vi "Is Point In Shape(1).vi"(8 "error in (no error)":errorcluster, 10 "Point":cluster{"Horizontal":i32, "Vertical":i32}, 11 "Rectangle in":refnum<class "Rectangle.lvclass">) -> (0 "error out":errorcluster, 2 "Point In Shape?":bool, 3 "Rectangle out":refnum<class "Rectangle.lvclass">)   [LabVIEW 2015, in "Rectangle.lvclass"]
uses:
  Rectangle.lvclass
  Interfaces/Shape/Shape.lvclass/Shape.ctl
  Interfaces/Shape/Shape.lvclass
panel:
  # "NOTICE -- YOU MUST LEAVE THIS NOTICE IN PLACE.\n\nCopyright (c) 2017, LIANG LIU Shawn.Liu.cn@gmail.com\nAll rights reserved.\n\nRedistribution and use in source and binary forms, with or without modification, are permitted provided that the following conditions are met:\n-Redistributions of source code must retain the above copyright notice, this list of conditions and the following disclaimer.\n-Redistributions in binary form must reproduce the above copyright notice, this list of conditions and the following disclaimer in the documentation and/or other materials provided with the distribution.\n-Neither the name of the eLp nor the names of its contributors may be used to endorse or promote products derived from this software without specific prior written permission.\n\nTHIS SOFTWARE IS PROVIDED BY THE COPYRIGHT HOLDERS AND CONTRIBUTORS \"AS IS\" AND ANY EXPRESS OR IMPLIED WARRANTIES, INCLUDING, BUT NOT LIMITED TO, THE IMPLIED WARRANTIES OF MERCHANTABILITY AND FITNESS FOR A PARTICULAR PURPOSE ARE DISCLAIMED. IN NO EVENT SHALL THE COPYRIGHT HOLDER OR CONTRIBUTORS BE LIABLE FOR ANY DIRECT, INDIRECT, INCIDENTAL, SPECIAL, EXEMPLARY, OR CONSEQUENTIAL DAMAGES (INCLUDING, BUT NOT LIMITED TO, PROCUREMENT OF SUBSTITUTE GOODS OR SERVICES; LOSS OF USE, DATA, OR PROFITS; OR BUSINESS INTERRUPTION) HOWEVER CAUSED AND ON ANY THEORY OF LIABILITY, WHETHER IN CONTRACT, STRICT LIABILITY, OR TORT (INCLUDING NEGLIGENCE OR OTHERWISE) ARISING IN ANY WAY OUT OF THE USE OF THIS SOFTWARE, EVEN IF ADVISED OF THE POSSIBILITY OF SUCH DAMAGE."
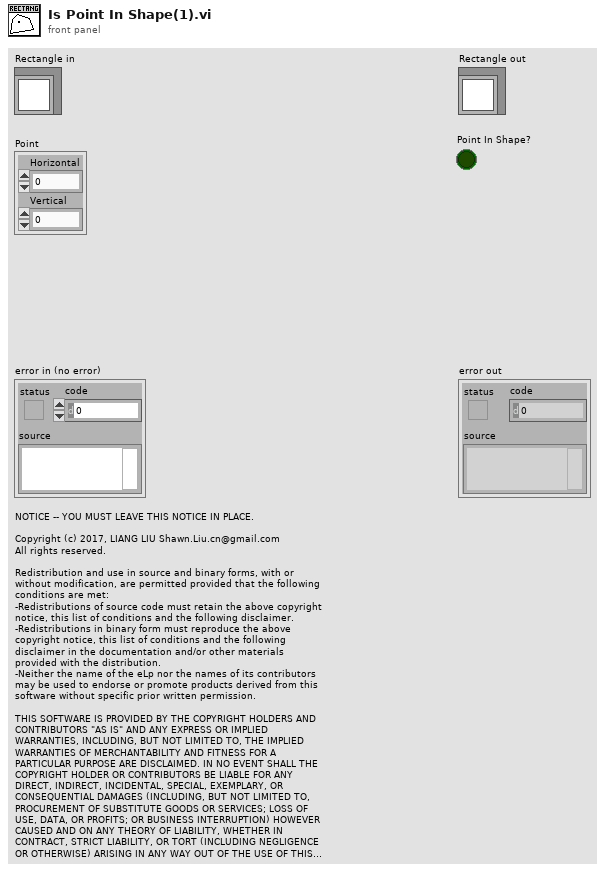
[diagram p1: front panel]
types:
  T1 = cluster{"left":i16, "top":i16, "right":i16, "bottom":i16}
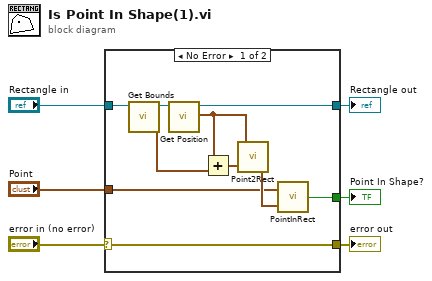
[diagram p0: block diagram]
diagram:
  n1 = case shown="No Error" "error in (no error)" {
    selector: "error in (no error)" -> [w16 w18]
    tunnel: "Rectangle in" -> [w15 w17]
    tunnel: [w13 w17] -> w4
    tunnel: "Point" -> [w8 _]
    tunnel: [w7 _] -> w2
    tunnel: [w16 w18] -> w1
    frame No Error {
      n2 = call "Get Bounds.vi"("Shape in"=w15) -> ("Bounds"=w11:cluster{"Width":u32, "Height":u32}, "Shape out"=w14:refnum<class "Rectangle.lvclass">)  [unwired: 9 in]
      n3 = call "Get Position.vi"("Shape in"=w14) -> ("Position"=w12:cluster{"Left":i32, "Top":i32}, "Shape out"=w13:refnum<class "Rectangle.lvclass">)  [unwired: 9 in]
      n4 = Add(x=w12, y=w11) -> (x+y=w10:cluster{u32, u32})
      n5 = call <vilib>:"Point2Rect.vi"("point b"=w10, "point a"=w12) -> ("rect"=w9:T1)
      n6 = call <vilib>:"PointInRect.vi"("rect"=w9, "point"=w8) -> ("pt in rect"=w7:bool)
    }
    frame Error {
    }
  }
  "error out" <- w1
  "Rectangle out" <- w4
  "Point In Shape?" <- w2
